vi "Write Memory.vi"(8 "error in (no error)":errorcluster, 9 "Memory Cell":T1, 10 "Memory Address":i32, 11 "gScript Interpreter in":refnum<class "gScript Interpreter.lvclass">) -> (0 "error out":errorcluster, 3 "gScript Interpreter out":refnum<class "gScript Interpreter.lvclass">)   [LabVIEW 2023, in "gScript Interpreter.lvclass"]
uses:
  gScript Interpreter.lvclass
  Type Definitions/Memory Cell.ctl
  Type Definitions/Memory Cell Type Enum.ctl
  gScript Interpreter.lvclass/gScript Interpreter.ctl
  <vilib>/Utility/error.llb/Error Cluster From Error Code.vi
  <vilib>/ErrorRing/Error Ring.xnode
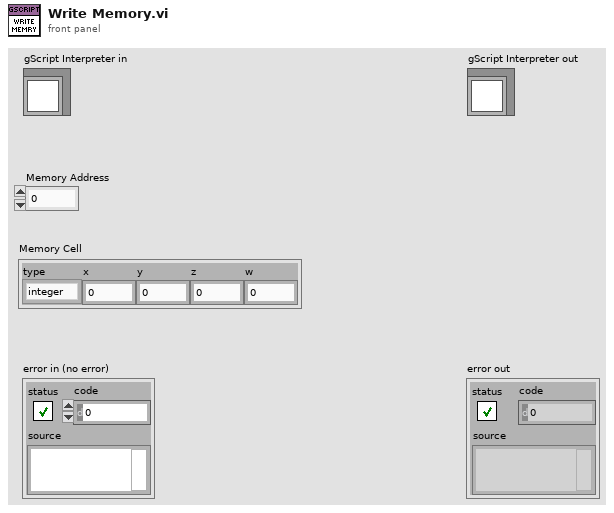
[diagram p1: front panel]
types:
  T1 = typedef "Memory Cell.ctl" = cluster{"type":T2, "x":dbl, "y":dbl, "z":dbl, "w":dbl}
  T2 = typedef "Memory Cell Type Enum.ctl" = enum16{"integer", "float", "vector", "rotation"}
  T3 = typedef "Main Memory.ctl" = T1[]
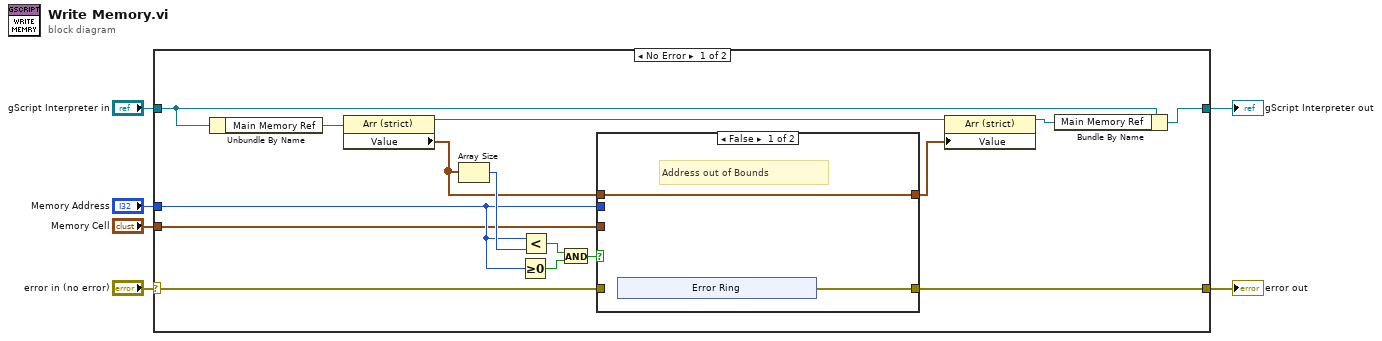
[diagram p0: block diagram]
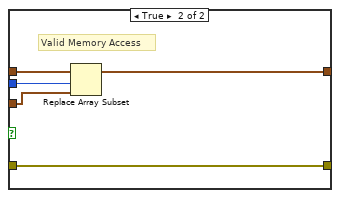
[diagram p2: hidden frame]
diagram:
  n1 = case shown="No Error" "error in (no error)" {
    selector: "error in (no error)" -> [w15 w34]
    tunnel: [w14 w34] -> w5
    tunnel: [w7 w33] -> w3
    tunnel: "gScript Interpreter in" -> [w9 w33]
    tunnel: "Memory Address" -> [w13 _]
    tunnel: "Memory Cell" -> [w12 _]
    frame No Error {
      n2 = Unbundle By Name(w9) -> ("Main Memory Ref"=w21:refnum<vi>)
      n3 = property class="Arr (strict)"(reference=w21) -> (reference out=w11:refnum<vi>, "Value"=w16:T3)  [unwired: 1 in, 1 out]
      n4 = Array Size(array=w16) -> (size(s)=w20:i32)
      n5 = Greater Or Equal To 0?(x=w13) -> (x >= 0?=w18:bool)
      n6 = Less?(x=w13, y=w20) -> (x < y?=w19:bool)
      n7 = And(x=w19, y=w18) -> (x .and. y?=w17:bool)
      n8 = case shown="False" w17 {
        tunnel: w16 -> [w22 w31]
        tunnel: [w22 w28] -> w10
        tunnel: w15 -> [_ w32]
        tunnel: [w23 w32] -> w14
        tunnel: w13 -> [_ w30]
        tunnel: w12 -> [_ w29]
        frame False {
          # "Address out of Bounds"
          n9 = xnode "Error Ring"() -> ("error out"=w23:errorcluster)
        }
        frame True {
          # "Valid Memory Access"
          n10 = Replace Array Subset(array=w31, new element=w29, index=w30) -> (w28:T3)
        }
      }
      n11 = property class="Arr (strict)"(reference=w11, "Value"=w10) -> (reference out=w8:refnum<vi>)  [unwired: 1 in, 1 out]
      n12 = Bundle By Name(cluster=w9, "Main Memory Ref"=w8) -> (w7:refnum<class "gScript Interpreter.lvclass">)
    }
    frame Error {
    }
  }
  "error out" <- w5
  "gScript Interpreter out" <- w3
